vi "FittedCurvePolynom.vi"() -> ()   [LabVIEW 2013]
panel:
  in  "FittedCurvePolynom":dbl[](array[numeric])
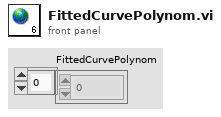
[diagram p1: front panel]
diagram:
